vi "test_Clear Slot.vi"(8 "error in (no error)":errorcluster, 11 "TestCase in":refnum<class "Scan Engine Scripting API Custom Device Unit Tests.lvclass">) -> (0 "error out":errorcluster, 3 "TestCase out":refnum<class "Scan Engine Scripting API Custom Device Unit Tests.lvclass">)   [LabVIEW 2019, in "Scan Engine Scripting API Custom Device Unit Tests.lvclass"]
uses:
  Scan Engine Scripting API Custom Device Unit Tests.lvclass
  <vilib>/addons/_JKI Toolkits/VI Tester/TestCase.llb/TestCase.lvclass
  Scripting/Scan Engine Scripting.lvlib
  Shared/Type Defs/Main Settings.ctl
  Shared/SEECD Shared.lvlib
  Shared/Type Defs/Local Chassis Settings.ctl
  Scripting/Modules/NI 9224/NI 9224.lvclass
  a134009e-d5c9-407c-b835-1c4aa24009a3.vi
  Scripting/Modules/Module/Module.lvclass
  C:/Users/nitest/Desktop/Git 2019/niveristand-scan-engine-ethercat-custom-device/Custom Device Source/Scripting/Modules/Module/Module.lvclass
  C:/Program Files (x86)/National Instruments/LabVIEW 2019/vi.lib/addons/_JKI Toolkits/VI Tester/TestCase.llb/TestCase.lvclass
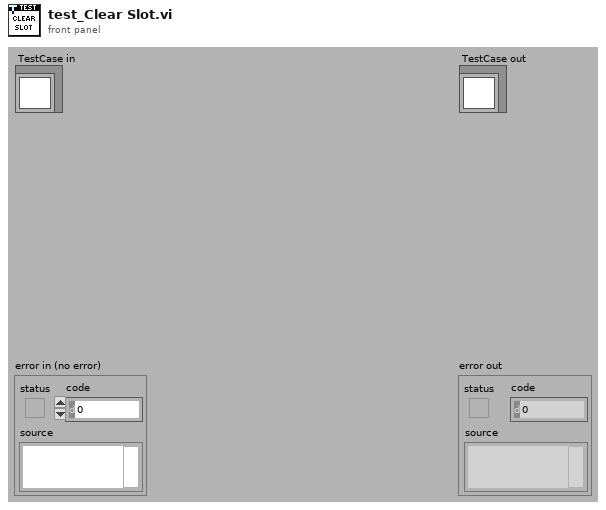
[diagram p1: front panel]
types:
  T1 = typedef "SEECD Shared.lvlib/Main Settings.ctl" = cluster{"sync to scan":bool, "scan engine decimation":u16, "delay after FPGA load (s)":u16}
  T2 = typedef "SEECD Shared.lvlib/Local Chassis Settings.ctl" = cluster{"name":string, "number of slots":i32}
  T3 = typedef "Custom Device API.lvlib/Custom Device Item Ref.ctl" = u64
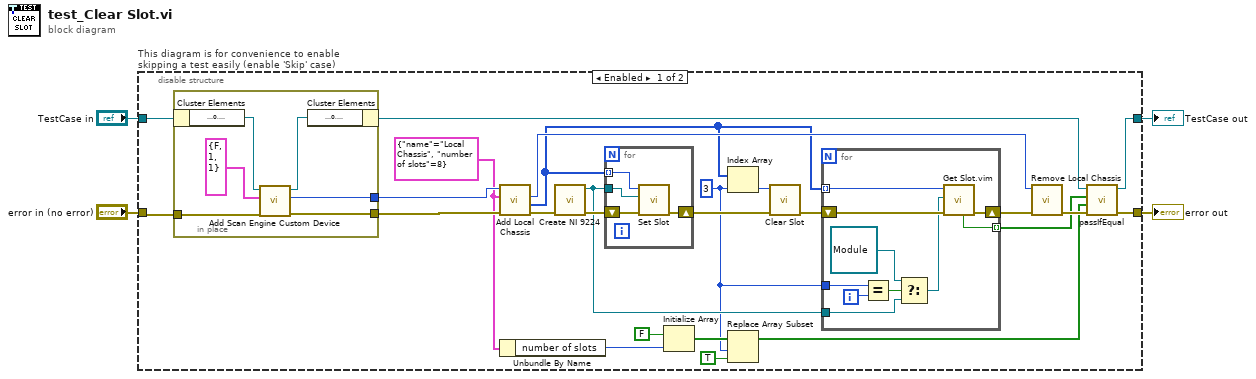
[diagram p0: block diagram]
diagram:
  n1 = disable-structure "This diagram is for convenience to enable skipping a test easily (enable 'Skip' case)" shown="Enabled" {
    disable-tunnel: "TestCase in" -> [w26 w53]
    disable-tunnel: [w9 w51] -> w1
    disable-tunnel: [w8 w52] -> w3
    disable-tunnel: "error in (no error)" -> [w27 w50]
    frame Enabled {
      w5 = 3 ("index")
      w13 = T2 {"name"="Local Chassis", "number of slots"=8} ("settings")
      n2 = in-place {
        in-place-border: [w35] -> w29
        in-place-border: [w34] -> w28
        in-place-border: w27 -> [w32]
        n3 = in-place-cluster #1(w26) -> ("target ref"=w31:refnum<k24>)
        n4 = call "Add Scan Engine Custom Device.vi"("error in"=w32, "settings"=T1 {"sync to scan"=FALSE, "scan engine decimation"=1, "delay after FPGA load (s)"=1}, "target in"=w31) -> ("error out"=w34:errorcluster, "scan engine custom device ref"=w35:T3, "target out"=w30:refnum<k24>)  [unwired: 6 in]
        n5 = in-place-cluster #1("target ref"=w30) -> (w25:refnum<class "Scan Engine Scripting API Custom Device Unit Tests.lvclass">)
      }
      n6 = call "Add Local Chassis.vi"("error in"=w28, "settings"=w13, "scan engine custom device ref in"=w29) -> ("error out"=w17:errorcluster, "slot refs"=w18:T3[], "local chassis ref"=w23:T3)  [unwired: 4 in, 2 out]
      n7 = Unbundle By Name(w13) -> ("number of slots"=w12:i32)
      n8 = call "Create NI 9224.vi"("error in"=w17) -> ("error out"=w16:errorcluster, "NI 9224 out"=w15:refnum<class "NI 9224.lvclass">)  [unwired: 9 in]
      n9 = for {
        tunnel: w18 -> [w48] mode=indexing
        shift-right: [w49] -> w22
        shift-left: w16 -> [w46]
        tunnel: w15 -> [w47]
        n10 = call "Set Slot.vi"("error in"=w46, "module"=w47, "slot ref in"=w48) -> ("error out"=w49:errorcluster)  [unwired: 7 in, 1 out]
      }
      n11 = Initialize Array(FALSE, w12) -> (w11:bool[])
      n12 = Index Array(array=w18, index=w5) -> (element=w21:T3)
      n13 = Replace Array Subset(array=w11, new element=TRUE, index=w5) -> (w7:bool[])
      n14 = call "Clear Slot.vi"("error in"=w22, "slot ref in"=w21) -> ("error out"=w20:errorcluster)  [unwired: 8 in, 1 out]
      n15 = for {
        shift-right: [w44] -> w19
        shift-left: w20 -> [w45]
        tunnel: w18 -> [w43] mode=indexing
        tunnel: w15 -> [w38]
        tunnel: [w42] -> w6 mode=indexing
        tunnel: w5 -> [w40]
        i -> [w39]
        n16 = Equal?(x=w40, y=w39) -> (x = y?=w41:bool)
        n17 = Select(t=refnum<class "Module.lvclass"> refnum ("Scan Engine Scripting.lvlib:Module.lvclass"), s=w41, f=w38) -> (s? t:f=w37:refnum<class "Module.lvclass">)
        n18 = call "Get Slot.vim"("error in"=w45, "module type"=w37, "slot ref in"=w43) -> ("error out"=w44:errorcluster, "empty"=w42:bool)  [unwired: 5 in, 2 out]
      }
      n19 = call "Remove Local Chassis.vi"("error in"=w19, "local chassis ref"=w23) -> ("error out"=w24:errorcluster)  [unwired: 9 in]
      n20 = call-dynamic "passIfEqual.vi"("error in (no error)"=w24, "y"=w7, "x"=w6, "TestCase in"=w25) -> ("error out"=w8:errorcluster, "TestCase out"=w9:refnum<class "Scan Engine Scripting API Custom Device Unit Tests.lvclass">)  [unwired: 6 in]
    }
    frame Disabled {
      # "skip test result while test is under development"
      n21 = call <vilib>:"skip.vi"("error in (no error)"=w50, "TestCase in"=w53) -> ("error out"=w52:errorcluster, "TestCase out"=w51:refnum<class "Scan Engine Scripting API Custom Device Unit Tests.lvclass">)  [unwired: 8 in]
    }
  }
  "error out" <- w3
  "TestCase out" <- w1
